vi "subGetBuildSpecificationRefByName.vi"(8 "error in (no error)":errorcluster, 9 "ProjectItem in":refnum<class "ProjectItem.lvclass">, 11 "BuildManager in":refnum<class "BuildManager.lvclass">) -> (0 "error out":errorcluster, 1 "Build spec ref":refnum<vi>, 3 "BuildManager out":refnum<class "BuildManager.lvclass">)   [LabVIEW 2019, in "SolutionBuilder.lvlib" / "BuildManager.lvclass"]
uses:
  BuildManager.lvclass
  ProjectItem/ProjectItem.lvclass
  ProjectItem/ProjectItem.lvclass/ProjectItem.ctl
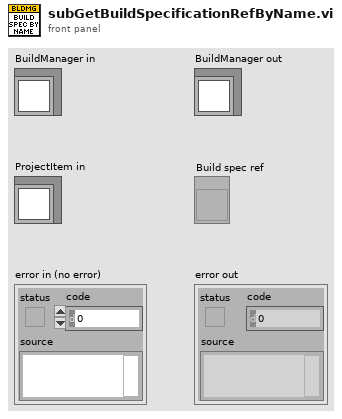
[diagram p1: front panel]
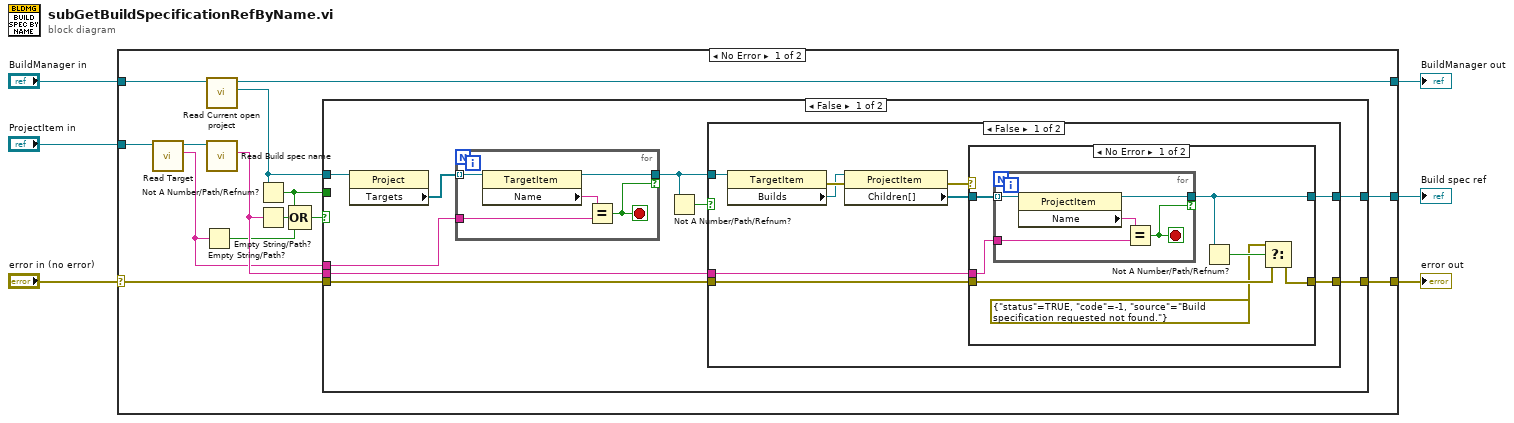
[diagram p0: block diagram]
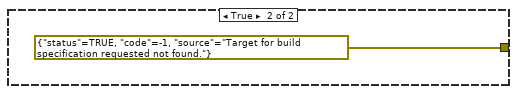
[diagram p3: hidden frame]
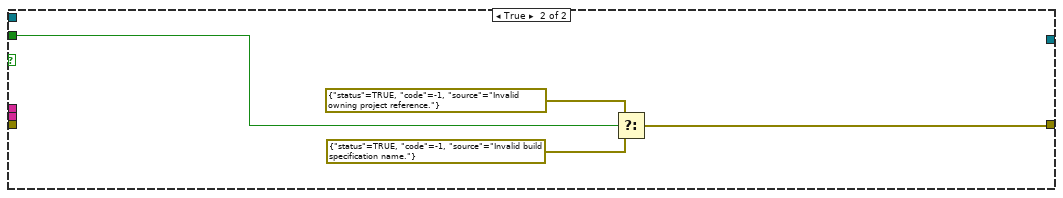
[diagram p4: hidden frame]
diagram:
  n1 = case shown="No Error" "error in (no error)" {
    selector: "error in (no error)" -> [w19 w63]
    tunnel: [w20 _] -> w6
    tunnel: [w18 w63] -> w4
    tunnel: "BuildManager in" -> [w7 w62]
    tunnel: [w14 w62] -> w2
    tunnel: "ProjectItem in" -> [w11 _]
    frame No Error {
      n2 = call "Read Target.vi"("ProjectItem in"=w11) -> ("Target"=w9:string, "ProjectItem out"=w10:refnum<class "ProjectItem.lvclass">)  [unwired: 9 in]
      n3 = Empty String/Path?(string/path=w9) -> (empty?=w8:bool)
      n4 = call-dynamic "Read Current open project.vi"("BuildManager in"=w7) -> ("Current open project"=w13:refnum<vi>, "BuildManager out"=w14:refnum<class "BuildManager.lvclass">)  [unwired: 9 in]
      n5 = call-dynamic "Read Build spec name.vi"("ProjectItem in"=w10) -> ("Build spec name"=w12:string)  [unwired: 9 in, 1 out]
      n6 = Not A Number/Path/Refnum?(number/path/refnum=w13) -> (NaN/Path/Refnum?=w15:bool)
      n7 = Empty String/Path?(string/path=w12) -> (empty?=w17:bool)
      n8 = Compound Arithmetic op=OR(w15, w17, w8) -> (w16:bool)
      n9 = case shown="False" w16 {
        tunnel: w12 -> [w29 _]
        tunnel: [w28 _] -> w20
        tunnel: w13 -> [w27 _]
        tunnel: w19 -> [w26 _]
        tunnel: [w25 w59] -> w18
        tunnel: w15 -> [_ w61]
        tunnel: w9 -> [w23 _]
        frame False {
          n10 = property class="Project"(reference=w27) -> ("Targets"=w24:refnum<vi>[])  [unwired: 1 in, 2 out]
          n11 = for {
            tunnel: w24 -> [w57] mode=indexing
            tunnel: w23 -> [w55]
            tunnel: [w54] -> w22 if=w53
            stop <- w53 stop-if-true
            n12 = property class="TargetItem"(reference=w57) -> (reference out=w54:refnum<vi>, "Name"=w56:string)  [unwired: 1 in, 1 out]
            n13 = Equal?(x=w56, y=w55) -> (x = y?=w53:bool)
          }
          n14 = Not A Number/Path/Refnum?(number/path/refnum=w22) -> (NaN/Path/Refnum?=w21:bool)
          n15 = case shown="False" w21 {
            tunnel: w29 -> [w35 _]
            tunnel: [w34 _] -> w28
            tunnel: w26 -> [w32 _]
            tunnel: [w31 errorcluster {"status"=TRUE, "code"=-1, "source"="Target for build specification requested not found."} ("t")] -> w25
            tunnel: w22 -> [w30 _]
            frame False {
              n16 = property class="TargetItem"(reference=w30) -> (error out=w38:errorcluster, "Builds"=w36:refnum<vi>)  [unwired: 1 in, 1 out]
              n17 = property class="ProjectItem"(reference=w36, error in=w38) -> (error out=w33:errorcluster, "Children[]"=w37:refnum<vi>[])  [unwired: 1 out]
              n18 = case shown="No Error" w33 {
                selector: w33 -> [_ w51]
                tunnel: w37 -> [w45 _]
                tunnel: w35 -> [w44 _]
                tunnel: [w43 _] -> w34
                tunnel: w32 -> [w41 _]
                tunnel: [w40 w51] -> w31
                frame No Error {
                  n19 = for {
                    tunnel: w45 -> [w50] mode=indexing
                    tunnel: w44 -> [w48]
                    tunnel: [w47] -> w43 if=w46
                    stop <- w46 stop-if-true
                    n20 = property class="ProjectItem"(reference=w50) -> (reference out=w47:refnum<vi>, "Name"=w49:string)  [unwired: 1 in, 1 out]
                    n21 = Equal?(x=w49, y=w48) -> (x = y?=w46:bool)
                  }
                  n22 = Not A Number/Path/Refnum?(number/path/refnum=w43) -> (NaN/Path/Refnum?=w42:bool)
                  n23 = Select(t=errorcluster {"status"=TRUE, "code"=-1, "source"="Build specification requested not found."}, s=w42, f=w41) -> (s? t:f=w40:errorcluster)
                }
                frame Error {
                }
              }
            }
            frame True {
            }
          }
        }
        frame True {
          n24 = Select(t=errorcluster {"status"=TRUE, "code"=-1, "source"="Invalid owning project reference."}, s=w61, f=errorcluster {"status"=TRUE, "code"=-1, "source"="Invalid build specification name."} ("t")) -> (s? t:f=w59:errorcluster)
        }
      }
    }
    frame Error {
    }
  }
  "error out" <- w4
  "BuildManager out" <- w2
  "Build spec ref" <- w6
